vi "ExOMAVStrip.vi"() -> ()   [LabVIEW 2010]
panel:
  out "Strip":sgl[](graph)
  in  "Temperature":dbl=-10.0 format="%.2f"
  in  "Exposure":dbl min=0.0 step=0.001 format="%.3f"
  in  "stop":bool
  out "error out":errorcluster
  in  "error in (no error)":errorcluster
  # "ExCenterStrip:\nThis example selects the center strip of the CCD for the ROI and then \ncollects the data using circular buffers. It collects data until the stop \nbutton is pushed."
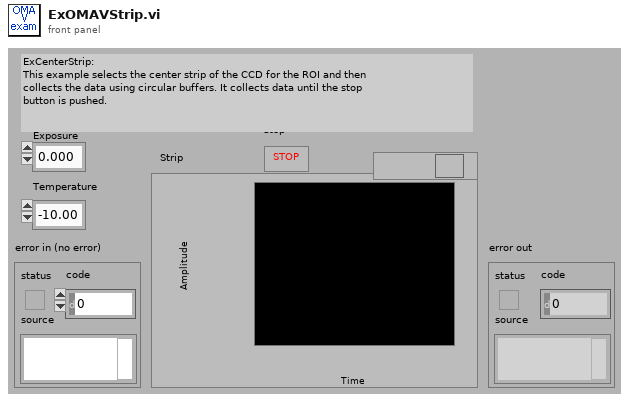
[diagram p1: front panel]
types:
  T1 = cluster{"Acquire / focus mode \n1 is Sync circualar buffers":i32, "Exposure":dbl, "Number of Images":i32, "Number of software\naccumulations":i32}
  T2 = cluster{"Camera Handle":u32, "Pulser Handle":u32, "File Handle":u32, "Display Handle":u32, "Image Handle":u32}
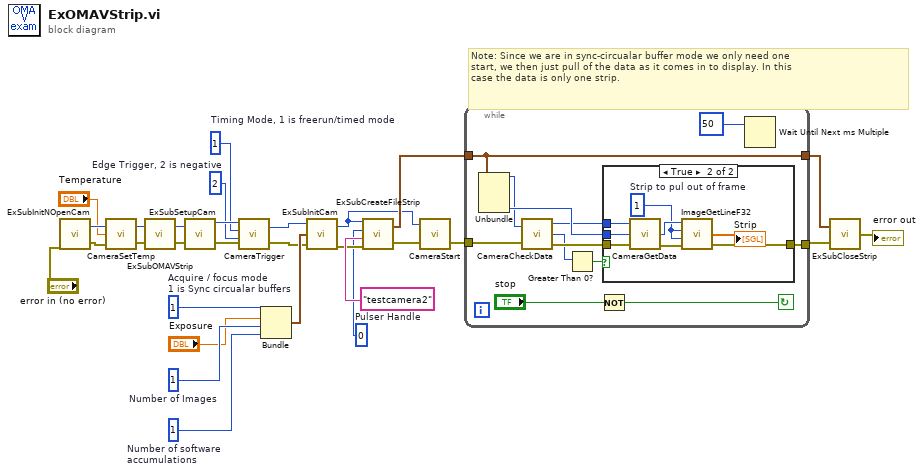
[diagram p0: block diagram]
diagram:
  w11 = 2  # Edge Trigger, 2 is negative
  w12 = 1  # Timing Mode, 1 is freerun/timed mode
  w21 = 0  # Pulser Handle
  w27 = 1  # Number of Images
  w28 = 1  # Acquire / focus mode  1 is Sync circualar buffers
  w26 = 1  # Number of software accumulations
  # "Note: Since we are in sync-circualar buffer mode we only need one\nstart, we then just pull of the data as it comes in to display. In this \ncase the data is only one strip."
  n1 = call "ExSubInitNOpenCam.vi"("error in (no error)"="error in (no error)") -> ("Camera Handle"=w3:u32, "error out"=w2:errorcluster)
  n2 = call <userlib>:"CameraSetTemp.vi"("error in (no error)"=w2, "Temperature"="Temperature", "Camera Handle"=w3) -> ("error out"=w4:errorcluster, "Camera Handle"=w5:u32)
  n3 = call "ExSubOMAVStrip.vi"("error in (no error)"=w4, "Camera Handle"=w5) -> ("error out"=w7:errorcluster, "Camera Handle"=w6:u32)
  n4 = call "ExSubSetupCam.vi"("error in (no error)"=w7, "Camera Handle"=w6) -> ("error out"=w10:errorcluster, "Camera Handle"=w14:u32)
  n5 = call <userlib>:"CameraTrigger.vi"("error in"=w10, "Trigger Edge"=w11, "Timing Mode"=w12, "Camera Handle"=w14) -> ("error out"=w15:errorcluster, "Camera Handle"=w13:u32)
  n6 = Bundle("Acquire / focus mode \n1 is Sync circualar buffers"=w28, "Exposure"="Exposure", "Number of Images"=w27, "Number of software\naccumulations"=w26) -> (w23:T1)  [unwired: 1 in]
  n7 = call "ExSubInitCam.vi"("error in (no error)"=w15, "Camera Information"=w23, "Camera Handle"=w13) -> ("error out"=w22:errorcluster, "Camera Handle"=w19:u32)
  n8 = call "ExSubCreateFileStrip.vi"("error in (no error)"=w22, "File and Display Name"="testcamera2", "Pulser Handle"=w21, "Camera Handle"=w19) -> ("error out"=w8:errorcluster, "Handles Out"=w20:T2)
  n9 = call <userlib>:"CameraStart.vi"("error in"=w8, "Camera Handle"=w19) -> ("error out"=w9:errorcluster)  [unwired: 1 out]
  n10 = while {
    tunnel: w20 -> [w38]
    tunnel: w9 -> [w37]
    tunnel: [w35] -> w17
    tunnel: [w38] -> w18
    stop <- w39 continue-if-true
    n11 = Unbundle(w38) -> ("Camera Handle"=w33:u32, "Image Handle"=w34:u32)  [unwired: 3 out]
    n12 = call <userlib>:"CameraCheckData.vi"("Camera Handle"=w33, "error in"=w37) -> ("Camera Handle"=w32:u32, "Number Of Frames Available"=w30:i32, "error out"=w36:errorcluster)
    n13 = Greater Than 0?(x=w30) -> (x > 0?=w31:bool)
    n14 = Not(x="stop") -> (.not. x?=w39:bool)
    n15 = case shown="True" w31 {
      tunnel: w36 -> [w42 w49]
      tunnel: [w42 w47] -> w35
      tunnel: w34 -> [_ w44]
      tunnel: w32 -> [_ w43]
      frame False {
      }
      frame True {
        w45 = 1  # Strip to pul out of frame
        n16 = call <userlib>:"CameraGetData.vi"("error in"=w49, "Data Handle"=w44, "Camera Handle"=w43) -> ("error out"=w48:errorcluster, "Data Handle"=w46:u32)  [unwired: 1 out]
        n17 = call <userlib>:"ImageGetLineF32.vi"("error in"=w48, "Z Position"=w45, "Y Position"=w45, "Data Handle"=w46) -> ("error out"=w47:errorcluster, "Array F32"=→"Strip":sgl[])  [unwired: 1 out]
      }
    }
    n18 = Wait Until Next ms Multiple(millisecond multiple=50) -> ()  [unwired: 1 out]
  }
  n19 = call "ExSubCloseStrip.vi"("error in (no error)"=w17, "Handles In"=w18) -> ("error out"=→"error out":errorcluster)
